vi "ZachArmPosition.vi"(8 "Manual Position":dbl, 9 "Arm Position":dbl, 11 "User Arm Position":T1) -> (1 "Target Position":dbl, 2 "Motor Speed":dbl)   [LabVIEW 2013]
uses:
  Arm Postions Enum Typedef.ctl
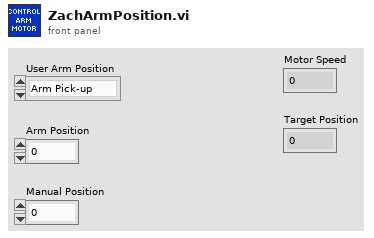
[diagram p1: front panel]
types:
  T1 = typedef "Arm Postions Enum Typedef.ctl" = enum16{"Arm Pick-up", "Arm Shoot", "Arm Truss", "Manual"}
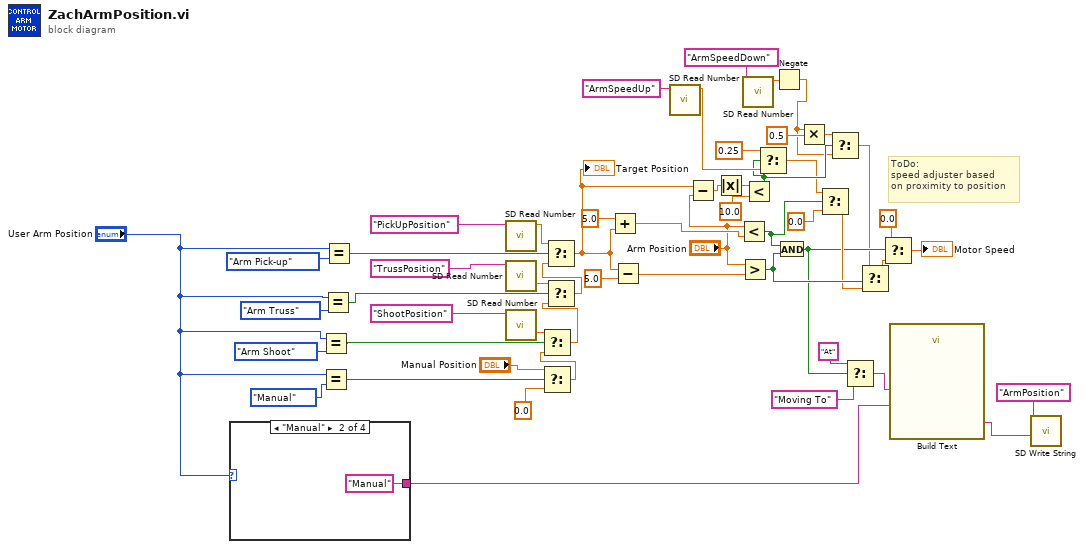
[diagram p0: block diagram]
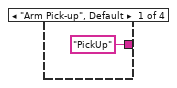
[diagram p2: hidden frame]
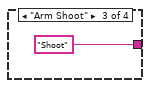
[diagram p3: hidden frame]
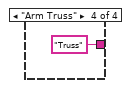
[diagram p4: hidden frame]
diagram:
  # "ToDo:\nspeed adjuster based\non proximity to position"
  n1 = case shown="\"Manual\"" "User Arm Position" {
    tunnel: ["PickUp" "Manual" "Shoot" "Truss"] -> w29
    frame "Arm Pick-up", Default {
    }
    frame "Manual" {
    }
    frame "Arm Shoot" {
    }
    frame "Arm Truss" {
    }
  }
  n2 = Equal?(x="User Arm Position", y=Arm_Postions_Enum_Typedef."Arm Shoot") -> (x = y?=w41:bool)
  n3 = Equal?(x="User Arm Position", y=Arm_Postions_Enum_Typedef."Manual") -> (x = y?=w4:bool)
  n4 = Equal?(x="User Arm Position", y=Arm_Postions_Enum_Typedef."Arm Truss") -> (x = y?=w42:bool)
  n5 = Equal?(x="User Arm Position", y=Arm_Postions_Enum_Typedef."Arm Pick-up") -> (x = y?=w40:bool)
  n6 = call <vilib>:"SD Read Number.vi"("Name"="PickUpPosition" ("Table Prefix")) -> ("Numeric"=w21:dbl)  [unwired: 8 in, 2 out]
  n7 = call <vilib>:"SD Read Number.vi"("Name"="TrussPosition" ("Table Prefix")) -> ("Numeric"=w35:dbl)  [unwired: 8 in, 2 out]
  n8 = call <vilib>:"SD Read Number.vi"("Name"="ShootPosition" ("Table Prefix")) -> ("Numeric"=w34:dbl)  [unwired: 8 in, 2 out]
  n9 = Select(t="Manual Position", s=w4, f=0.0) -> (s? t:f=w6:dbl)
  n10 = Select(t=w34, s=w41, f=w6) -> (s? t:f=w53:dbl)
  n11 = Select(t=w35, s=w42, f=w53) -> (s? t:f=w54:dbl)
  n12 = Select(t=w21, s=w40, f=w54) -> (s? t:f=w2:dbl)
  "Target Position" <- w2
  n13 = Add(x=5.0, y=w2) -> (x+y=w49:dbl)
  n14 = Subtract(x=w2, y=5.0) -> (x-y=w50:dbl)
  n15 = call <vilib>:"SD Read Number.vi"("Name"="ArmSpeedUp") -> ("Numeric"=w20:dbl)  [unwired: 8 in, 2 out]
  n16 = Subtract(x=w2, y="Arm Position") -> (x-y=w17:dbl)
  n17 = Absolute Value(x=w17) -> (abs(x)=w16:dbl)
  n18 = Less?(x="Arm Position", y=w49) -> (x < y?=w48:bool)
  n19 = Greater?(x="Arm Position", y=w50) -> (0:w47:bool)
  n20 = call <vilib>:"SD Read Number.vi"("Name"="ArmSpeedDown") -> ("Numeric"=w10:dbl)  [unwired: 8 in, 2 out]
  n21 = Less?(x=w16, y=10.0) -> (x < y?=w13:bool)
  n22 = Select(t=0.25, s=w13, f=w20) -> (s? t:f=w11:dbl)
  n23 = Negate(x=w10) -> (-x=w9:dbl)
  n24 = And(x=w48, y=w47) -> (x .and. y?=w25:bool)
  n25 = Multiply(x=w9, y=0.5) -> (x*y=w19:dbl)
  n26 = Select(t=w11, s=w48, f=0.0) -> (s? t:f=w46:dbl)
  n27 = Select(t=w19, s=w13, f=w9) -> (s? t:f=w12:dbl)
  n28 = Select(t="At" ("Name"), s=w25, f="Moving To" ("Name")) -> (s? t:f=w28:string)
  n29 = Select(t=w12, s=w47, f=w46) -> (s? t:f=w45:dbl)
  n30 = Select(t=0.0, s=w25, f=w45) -> (s? t:f=→"Motor Speed":dbl)
  n31 = call "Build Text"("Moving"=w28, "Place"=w29) -> ("Result"=w33:string)  [unwired: 12 in, 1 out]
  n32 = call <vilib>:"SD Write String.vi"("String"=w33, "Name"="ArmPosition") -> ()  [unwired: 8 in, 2 out]
